vi "Script Logging.vi"(8 "error in (no error)":errorcluster, 11 "Ballard MIL-STD 1553 custom device in":T1 format="%.0x") -> (0 "error out":errorcluster, 2 "RT log file path":string, 3 "Ballard MIL-STD 1553 custom device out":T1 format="%.0x")   [LabVIEW 2020, in "Logging Loopback.lvclass"]
uses:
  Logging Loopback.lvclass
  Scripting/AIM MIL-STD-1553 Scripting.lvlib
  <vilib>/NI VeriStand/Custom Device API/Custom Device Item Ref.ctl
  <vilib>/NI VeriStand/Custom Device API/Custom Device API.lvlib
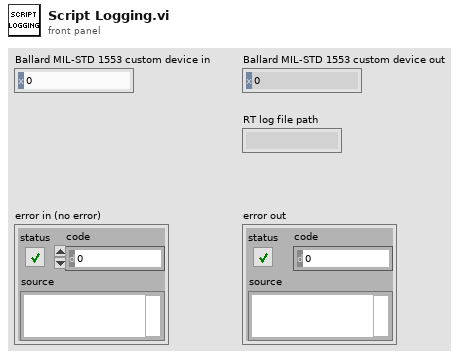
[diagram p1: front panel]
types:
  T1 = typedef "Custom Device API.lvlib/Custom Device Item Ref.ctl" = u64
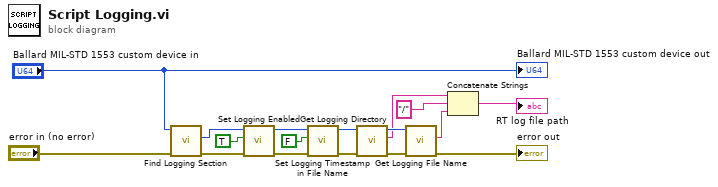
[diagram p0: block diagram]
diagram:
  n1 = call "Find Logging Section.vi"("error in"="error in (no error)", "Ballard MIL-STD 1553 custom device in"="Ballard MIL-STD 1553 custom device in") -> ("error out"=w9:errorcluster, "logging"=w13:T1)  [unwired: 7 in, 1 out]
  n2 = call "Set Logging Enabled.vi"("error in"=w9, "logging enabled"=TRUE, "logging in"=w13) -> ("error out"=w8:errorcluster, "logging out"=w11:T1)  [unwired: 7 in]
  n3 = call "Set Logging Timestamp in File Name.vi"("error in"=w8, "timestamp in file name"=FALSE, "logging in"=w11) -> ("error out"=w6:errorcluster, "logging out"=w7:T1)  [unwired: 7 in]
  n4 = call "Get Logging Directory.vi"("error in"=w6, "logging in"=w7) -> ("error out"=w15:errorcluster, "directory"=w3:string, "logging out"=w14:T1)  [unwired: 7 in]
  n5 = call "Get Logging File Name.vi"("error in"=w15, "logging in"=w14) -> ("error out"=→"error out":errorcluster, "file name"=w2:string)  [unwired: 7 in, 1 out]
  n6 = Concatenate Strings(w3, "/" ("string"), w2) -> (→"RT log file path":string)
  "Ballard MIL-STD 1553 custom device out" <- "Ballard MIL-STD 1553 custom device in"
